vi "Drive Angle Magnitude.vi"(8 "error in":errorcluster, 10 "data":variant=variant(cluster{"Angle":dbl, "Drive Magnitude":dbl, "Get ms ago":u32} {"Angle"=30.0, "Drive Magnitude"=0.0, "Get ms ago"=0}), 11 "DriveRef":T1={"queue"=refnum, "Drivetrain"={"DevStatus"={"status"=FALSE, "code"=0, "source"=""}, "Motors[]"=[{"DeviceStatus"={"status"=FALSE, "code"=0, "source"=""}, "Type"=enum."PWM", "PWM"={"PWM Channel"=enum."PWM 1", "DeadBand"={"Name"="SPARK", "maxPositivePwm"=1500, "minPositivePwm"=1010, "centerPwm"=1005, "maxNegativePwm"=1000, "minNegativePwm"=500, "angularRange"=0}}, "CAN"={"Device Number"=0, "SetOutput VI Ref"=variant(refnum<vi> refnum), "GetOutput VI Ref"=variant(refnum<vi> refnum), "Enable VI Ref"=variant(refnum<vi> refnum), "Disable VI Ref"=variant(refnum<vi> refnum), "Data"=variant}, "Invert"=TRUE}, {"DeviceStatus"={"status"=FALSE, "code"=0, "source"=""}, "Type"=enum."PWM", "PWM"={"PWM Channel"=enum."PWM 0", "DeadBand"={"Name"="SPARK", "maxPositivePwm"=1500, "minPositivePwm"=1010, "centerPwm"=1005, "maxNegativePwm"=1000, "minNegativePwm"=500, "angularRange"=0}}, "CAN"={"Device Number"=0, "SetOutput VI Ref"=variant(refnum<vi> refnum), "GetOutput VI Ref"=variant(refnum<vi> refnum), "Enable VI Ref"=variant(refnum<vi> refnum), "Disable VI Ref"=variant(refnum<vi> refnum), "Data"=variant}, "Invert"=FALSE}], "Square Inputs"=TRUE, "Max Output"=1.0}, "Encoder L"={"DevStatus"={"status"=FALSE, "code"=0, "source"=""}, "EncoderIndex"=enum."Enc 0", "CounterIndex"=enum."Invalid", "DistancePerCount"=0.0490874, "Decoding Type"=enum."4x"}, "Encoder R"={"DevStatus"={"status"=FALSE, "code"=0, "source"=""}, "EncoderIndex"=enum."Enc 1", "CounterIndex"=enum."Invalid", "DistancePerCount"=0.0490874, "Decoding Type"=enum."4x"}, "Gyro"={"DevStatus"={"status"=FALSE, "code"=0, "source"=""}, "Analog Channel"=enum."AI 1", "Offset"=0.0, "Gain (VoltsPerDegree/Second)"=0.0, "Gyro Type"=enum."XRS450", "Handle"=44, "SPI Bus"=enum."SPI On-Board, CS0", "Device Found"=TRUE, "Sample Rate"=1.0, "Calibrate On Open"=FALSE}, "Lock"={"notifier out"=refnum}, "Shifter"={"DevStatus"={"status"=FALSE, "code"=0, "source"=""}, "Pneumatics Control Module"=1, "Forward Solenoid Channel"=enum."Solenoid 0", "Reverse Solenoid Channel"=enum."Solenoid 1"}} {"Gyro"."Sample Rate" min=0.25 max=100.0 step=0.25}) -> (0 "error out":errorcluster)   [LabVIEW 2016, in "Drive System.lvlib"]
uses:
  Drive System.lvlib
  DriveMainType.ctl
  DriveCmd.ctl
  DriveCmdList.ctl
  <vilib>/Rock Robotics/WPI/RobotDrive/WPI_RobotDriveDevRef.ctl
  <vilib>/Rock Robotics/WPI/MotorControl/WPI_MotorControlDeviceRef.ctl
  <vilib>/Rock Robotics/WPI/MotorControl/WPI_MotorControlType.ctl
  <vilib>/Rock Robotics/SystemInterfaces/DIO/FPGA_DIOPWMChannel.ctl
  <vilib>/Rock Robotics/WPI/PWM/WPI_PWMDeadband.ctl
  <vilib>/Rock Robotics/WPI/Encoder/WPI_EncoderDevRef.ctl
  <vilib>/Rock Robotics/SystemInterfaces/Encoder/FPGA_EncoderIdx.ctl
  <vilib>/Rock Robotics/SystemInterfaces/Counter/FPGA_CounterCtrSystemIndex.ctl
  <vilib>/Rock Robotics/WPI/Encoder/WPI_EncoderType.ctl
  <vilib>/Rock Robotics/WPI/Gyro/WPI_GyroDevRef.ctl
  <vilib>/Rock Robotics/SystemInterfaces/AI/FPGA_AIChannel.ctl
  <vilib>/Rock Robotics/SystemInterfaces/spilib/spi_bus.ctl
  Varient Cmd Types/Lock Command.ctl
  <vilib>/Rock Robotics/WPI/Solenoid/WPI_SolenoidDevRef.ctl
  <vilib>/Rock Robotics/WPI/Solenoid/WPI_SolenoidChannel.ctl
  Varient Cmd Types/Drive Angle Magnitude.ctl
  <vilib>/Platform/TimedLoop/XDataNode/timing_clust.ctl
  <vilib>/Platform/TimedLoop/XDataNode/nitl_modes.ctl
  <vilib>/Platform/TimedLoop/XDataNode/wakeup.ctl
  <vilib>/Platform/TimedLoop/XDataNode/XDataNode.xnode
  <vilib>/Platform/TimedLoop/XDataNode/XDNodeRunTimeDep.lvlib
  Path Track/Path Track.lvlib
panel:
  out "Waveform Chart":cluster{"Drive Magnitude":dbl, "output":dbl}(graph)={"Drive Magnitude"=0.0, "output"=0.0009887805750059186}
  in  "PIDF gains":cluster{"Kp":dbl, "Ki":dbl, "Kd":dbl, "Kf":dbl}={"Kp"=0.0058, "Ki"=0.0, "Kd"=0.0155, "Kf"=0.0} {"Kf" format="%.3f"; "Kd" format="%.5f"; "Ki" format="%.5f"; "Kp" format="%.5f"}
  in  "i Zone":dbl=10.0 format="%.2f"
  # "Analog"
  # "XRS"
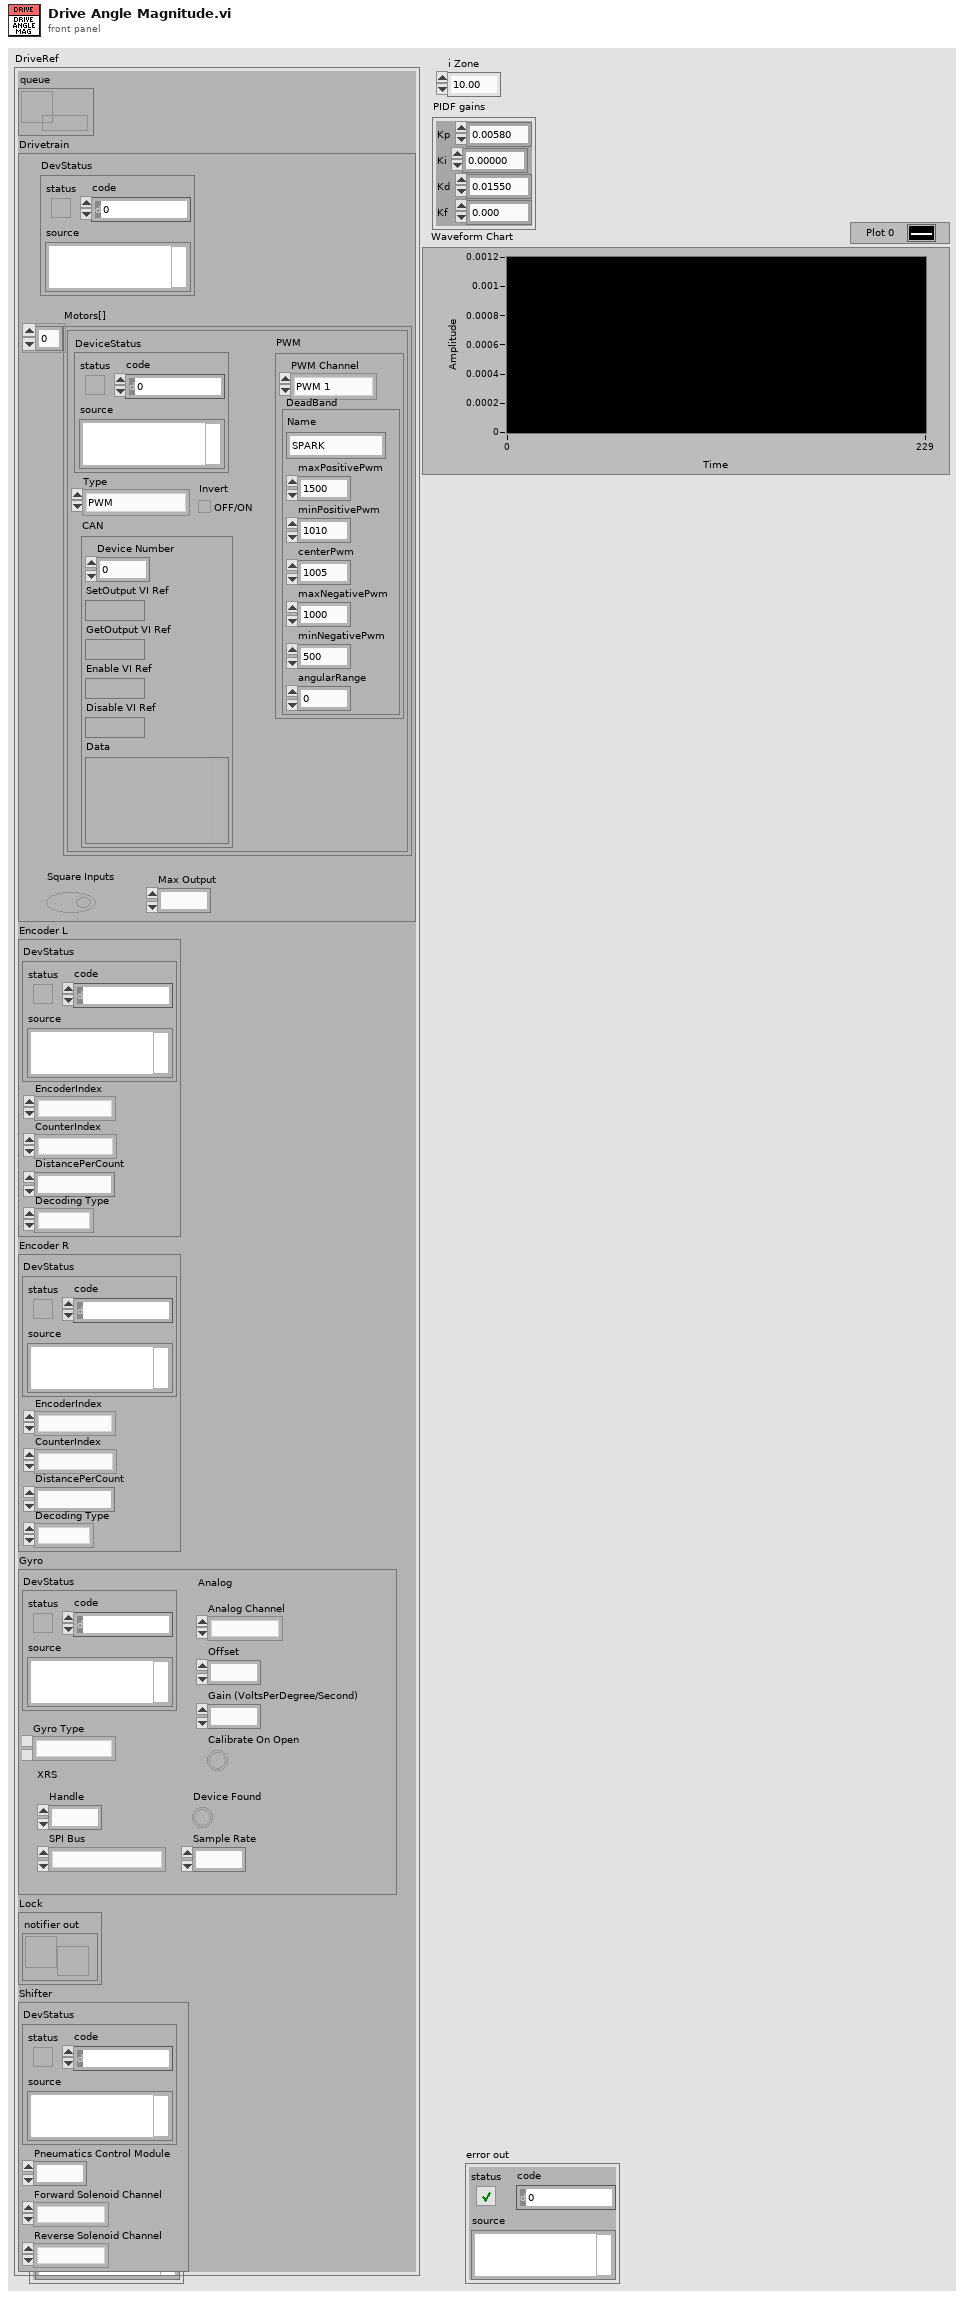
[diagram p1: front panel]
types:
  T1 = typedef "Drive System.lvlib/DriveMainType.ctl" = cluster{"queue":refnum<queue>, "Drivetrain":T2, "Encoder L":T7, "Encoder R":T7, "Gyro":T11, "Lock":T14, "Shifter":T15}
  T2 = typedef "WPI_RobotDriveDevRef.ctl" = cluster{"DevStatus":errorcluster, "Motors[]":T3[], "Square Inputs":bool, "Max Output":dbl}
  T3 = typedef "WPI_MotorControlDeviceRef.ctl" = cluster{"DeviceStatus":errorcluster, "Type":T4, "PWM":cluster{"PWM Channel":T5, "DeadBand":T6}, "CAN":cluster{"Device Number":u8, "SetOutput VI Ref":variant, "GetOutput VI Ref":variant, "Enable VI Ref":variant, "Disable VI Ref":variant, "Data":variant}, "Invert":bool}
  T4 = typedef "WPI_MotorControlType.ctl" = enum16{"PWM", "CAN"}
  T5 = typedef "FPGA_DIOPWMChannel.ctl" = enum8{"PWM 0", "PWM 1", "PWM 2", "PWM 3", "PWM 4", "PWM 5", "PWM 6", "PWM 7", "PWM 8", "PWM 9", "PWM MXP 0", "PWM MXP 1", "PWM MXP 2", "PWM MXP 3", "PWM MXP 4", "PWM MXP 5", "PWM MXP 6", "PWM MXP 7", "PWM MXP 8", "PWM MXP 9", "Invalid"}
  T6 = typedef "WPI_PWMDeadband.ctl" = cluster{"Name":string, "maxPositivePwm":i32, "minPositivePwm":i32, "centerPwm":i32, "maxNegativePwm":i32, "minNegativePwm":i32, "angularRange":u16}
  T7 = typedef "WPI_EncoderDevRef.ctl" = cluster{"DevStatus":errorcluster, "EncoderIndex":T8, "CounterIndex":T9, "DistancePerCount":dbl, "Decoding Type":T10}
  T8 = typedef "FPGA_EncoderIdx.ctl" = enum8{"Enc 0", "Enc 1", "Enc 2", "Enc 3", "Enc 4", "Enc 5", "Enc 6", "Enc 7", "Invalid"}
  T9 = typedef "FPGA_CounterCtrSystemIndex.ctl" = enum8{"Ctr 0", "Ctr 1", "Ctr 2", "Ctr 3", "Ctr 4", "Ctr 5", "Ctr 6", "Ctr 7", "Invalid"}
  T10 = typedef "WPI_EncoderType.ctl" = enum16{"1x", "2x", "4x"}
  T11 = typedef "WPI_GyroDevRef.ctl" = cluster{"DevStatus":errorcluster, "Analog Channel":T12, "Offset":dbl, "Gain (VoltsPerDegree/Second)":dbl, "Gyro Type":enum16{"Analog", "XRS450"}, "Handle":i32, "SPI Bus":T13, "Device Found":bool, "Sample Rate":dbl, "Calibrate On Open":bool}
  T12 = typedef "FPGA_AIChannel.ctl" = enum8{"AI 0", "AI 1", "AI 2", "AI 3", "AI MXP 0", "AI MXP 1", "AI MXP 2", "AI MXP 3", "Invalid"}
  T13 = typedef "spi_bus.ctl" = enum16{"SPI On-Board, CS0", "SPI On-Board, CS1", "SPI On-Board, CS2", "SPI On-Board, CS3", "SPI MXP", "Invalid"}
  T14 = typedef "Drive System.lvlib/Lock Command.ctl" = cluster{"notifier out":refnum<notifier>}
  T15 = typedef "WPI_SolenoidDevRef.ctl" = cluster{"DevStatus":errorcluster, "Pneumatics Control Module":u8, "Forward Solenoid Channel":T16, "Reverse Solenoid Channel":T16}
  T16 = typedef "WPI_SolenoidChannel.ctl" = enum8{"Solenoid 0", "Solenoid 1", "Solenoid 2", "Solenoid 3", "Solenoid 4", "Solenoid 5", "Solenoid 6", "Solenoid 7", "Invalid"}
  T17 = typedef "Drive System.lvlib/Drive Angle Magnitude.ctl" = cluster{"Angle":dbl, "Drive Magnitude":dbl, "Get ms ago":u32}
  T18 = typedef "XDNodeRunTimeDep.lvlib/timing_clust.ctl" = cluster{"Expected End [f-1]":u64, "Actual End [f-1]":u64, "Finished Late? [f-1]":bool, "Expected End [i-1]":u64, "Actual End [i-1]":u64, "Finished Late? [i-1]":bool, "Expected Start [i]":u64, "Actual Start [i]":u64, "Expected Start [f]":u64, "Actual Start [f]":u64, "Source Name":string, "Structure Name":string, "Period":i64, "Deadline":i64, "Offset":i64, "Start":i64, "Priority":i32, "Timeout":i32, "Mode":T19, "Wakeup Reason":T20, "Error":errorcluster, "Source Type":string, "Secondary Source Type":string, "Global End Time":u64, "Global Start Time":u64, "Frame Duration":u64, "Iteration Duration":u64, "Assigned CPU":i32, "I/O Scan Engine Mode":u32}
  T19 = typedef "XDNodeRunTimeDep.lvlib/nitl_modes.ctl" = enum32{"No Change", "Process missed periods, maintain original phase", "Discard missed periods, maintain original phase", "Process missed periods, ignore original phase", "Discard missed periods, ignore original phase"}
  T20 = typedef "XDNodeRunTimeDep.lvlib/wakeup.ctl" = enum32{"Normal", "Aborted", "Asynchronous wakeup", "Timing source error", "Timed loop error", "Timeout"}
  T21 = typedef "Drive System.lvlib/DriveCmd.ctl" = cluster{"cmd":T22, "data":variant, "Force? (F)":bool, "Lock":string}
  T22 = typedef "Drive System.lvlib/DriveCmdList.ctl" = enum16{"Idle", "Cleanup", "Drive For Time", "Follow Path Speed Control", "Follow Path", "Drive Tank", "Drive Straight PID", "Drive Angle Mag", "Drive Arcade", "Drive Ref", "Unlock", "Lock"}
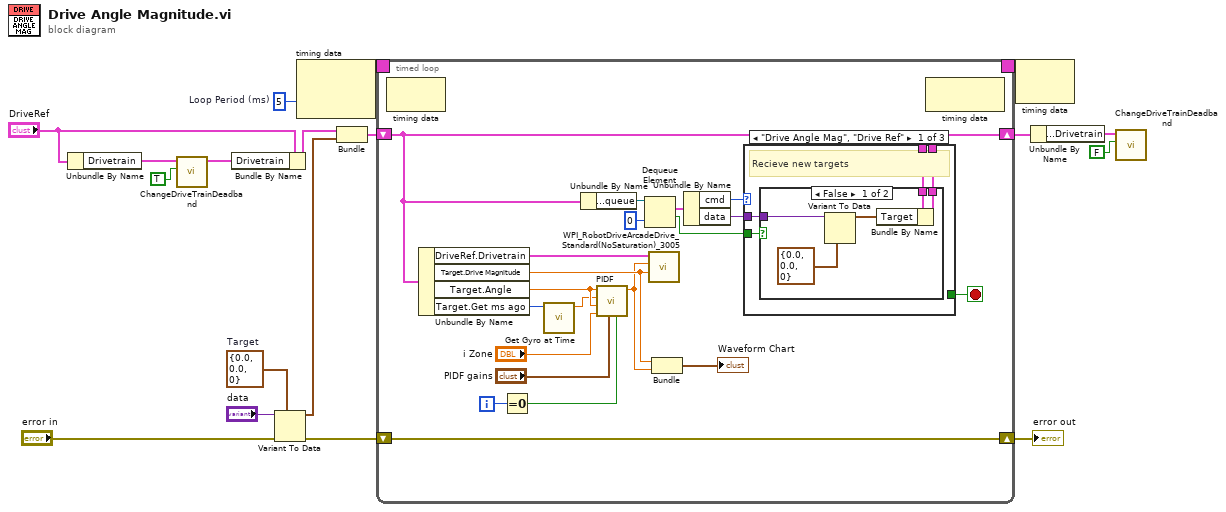
[diagram p0: block diagram]
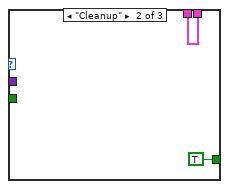
[diagram p3: hidden frame]
diagram:
  w2 = i64 5  # Loop Period (ms)
  w4 = T17 {"Angle"=0.0, "Drive Magnitude"=0.0, "Get ms ago"=0}  # Target
  n1 = Unbundle By Name("DriveRef") -> ("Drivetrain"=w11:T2)
  n2 = call "ChangeDriveTrainDeadband.vi"("Eliminate Deadband"=TRUE, "Drivetrain in"=w11) -> ("Drivetrain out"=w8:T2)  [unwired: 9 in]
  n3 = Bundle By Name(cluster="DriveRef", "Drivetrain"=w8) -> (w9:T1)
  n4 = Variant To Data(error in="error in", type=w4, Variant="data") -> (data=w3:T17, error out=w15:errorcluster)
  n5 = node-c288(w2) -> (w13:T18)  [unwired: 1 in]
  n6 = Bundle("DriveRef"=w9, "Target"=w3) -> (w17:cluster{"DriveRef":T1, "Target":T17})  [unwired: 1 in]
  n7 = timed-loop {
    shift-right: [w38] -> w18
    shift-left: w15 -> [w38]
    shift-right: [w31] -> w6
    shift-left: w17 -> [w30]
    timing: w13 -> [_]
    timing-out: [_] -> w12
    i -> [w25]
    stop <- w33 stop-if-true
    n8 = node-c288() -> ()  [unwired: 1 in, 1 out]
    n9 = Unbundle By Name(w30) -> ("DriveRef.Drivetrain"=w29:T2, "Target.Drive Magnitude"=w21:dbl, "Target.Angle"=w28:dbl, "Target.Get ms ago"=w22:u32)
    n10 = Equal To 0?(x=w25) -> (x = 0?=w24:bool)
    n11 = call "Get Gyro at Time.vi"("Get ms ago"=w22) -> ("Angle"=w23:dbl)  [unwired: 9 in, 1 out]
    n12 = Unbundle By Name(w30) -> ("DriveRef.queue"=w39:refnum<queue>)
    n13 = call "PIDF.vi"("reinitialize? (F)"=w24, "PIDF gains"="PIDF gains", "i Zone"="i Zone", "Feedforward"=w28, "process variable"=w23, "setpoint"=w28) -> ("output"=w20:dbl)  [unwired: 3 in, 2 out]
    n14 = Dequeue Element(queue=w39, timeout in ms (-1)=0) -> (element=w37:T21, timed out?=w34:bool)  [unwired: 1 in, 2 out]
    n15 = call "WPI_RobotDriveArcadeDrive_Standard(NoSaturation)_3005.vi"("Y axis value"=w21, "X axis value"=w20, "RobotDriveDevRef"=w29) -> ()  [unwired: 7 in, 2 out]
    n16 = Bundle("Drive Magnitude"=w21, "output"=w20) -> (→"Waveform Chart":cluster{"Drive Magnitude":dbl, "output":dbl})  [unwired: 1 in]
    n17 = Unbundle By Name(w37) -> ("cmd"=w35:T22, "data"=w32:variant)
    n18 = case shown="\"Drive Angle Mag\", \"Drive Ref\"" w35 {
      tunnel: w34 -> [w42 _ _]
      tunnel: [_ TRUE _] -> w33
      tunnel: w32 -> [w43 _ _]
      tunnel: [w41 w50 w52] -> w31
      tunnel: w30 -> [w40 w50 w52]
      frame "Drive Angle Mag", "Drive Ref" {
        # "Recieve new targets"
        n19 = case shown="False" w42 {
          tunnel: w43 -> [w47 _]
          tunnel: [w46 w49] -> w41
          tunnel: w40 -> [w45 w49]
          frame False {
            n20 = Variant To Data(type=T17 {"Angle"=0.0, "Drive Magnitude"=0.0, "Get ms ago"=0}, Variant=w47) -> (data=w44:T17)  [unwired: 1 in, 1 out]
            n21 = Bundle By Name(cluster=w45, "Target"=w44) -> (w46:cluster{"DriveRef":T1, "Target":T17})
          }
          frame True {
          }
        }
      }
      frame "Cleanup" {
      }
      frame Default {
      }
    }
    n22 = node-c288() -> ()  [unwired: 1 in, 1 out]
  }
  "error out" <- w18
  n23 = node-c288(w12) -> ()  [unwired: 1 out]
  n24 = Unbundle By Name(w6) -> ("DriveRef.Drivetrain"=w5:T2)
  n25 = call "ChangeDriveTrainDeadband.vi"("Eliminate Deadband"=FALSE, "Drivetrain in"=w5) -> ()  [unwired: 9 in, 1 out]
